vi "表配置.vi"(7 "Item":string, 8 "error in (no error)":errorcluster caption="错误输入（无错误）", 10 "Arguments":string[](array[string]), 11 "数字多用表接口输入":refnum<class "数字多用表接口.lvclass">) -> (0 "error out":errorcluster caption="错误输出", 3 "数字多用表接口输出":refnum<class "数字多用表接口.lvclass">)   [LabVIEW 2020]
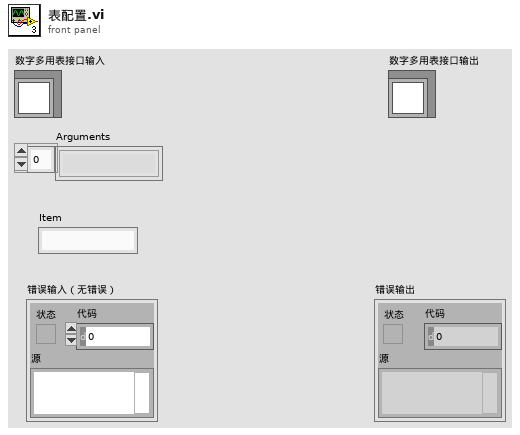
[diagram p1: front panel]
types:
  T1 = enum16{"DC Voltage", "AC Voltage", "Resistance", "DC Current", "AC Current"}
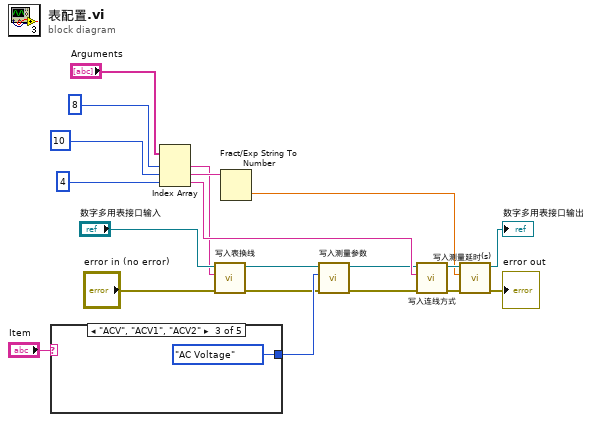
[diagram p0: block diagram]
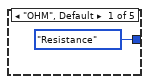
[diagram p2: hidden frame]
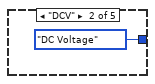
[diagram p3: hidden frame]
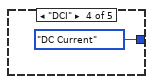
[diagram p4: hidden frame]
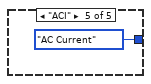
[diagram p5: hidden frame]
diagram:
  n1 = case shown="\"ACV\", \"ACV1\", \"ACV2\"" "Item" {
    tunnel: [T1."Resistance" ("测量参数") T1."DC Voltage" ("测量参数") T1."AC Voltage" ("测量参数") T1."DC Current" ("测量参数") T1."AC Current" ("测量参数")] -> w13
    frame "OHM", Default {
    }
    frame "DCV" {
    }
    frame "ACV", "ACV1", "ACV2" {
    }
    frame "DCI" {
    }
    frame "ACI" {
    }
  }
  n2 = Index Array(array="Arguments", index #1=8 ("索引"), index #2=10 ("索引"), index #3=4 ("索引")) -> (element #1=w4:string, element #2=w7:string, element #3=w15:string)
  n3 = call "写入表换线.vi"("error in (no error)"="error in (no error)", "表换线"=w4, "数字多用表接口输入"="数字多用表接口输入") -> ("error out"=w12:errorcluster, "数字多用表接口输出"=w16:refnum<class "数字多用表接口.lvclass">)  [unwired: 7 in]
  n4 = Fract/Exp String To Number(string=w7) -> (number=w6:dbl)  [unwired: 3 in, 1 out]
  n5 = call "写入测量参数.vi"("error in (no error)"=w12, "测量参数"=w13, "数字多用表接口输入"=w16) -> ("error out"=w10:errorcluster, "数字多用表接口输出"=w11:refnum<class "数字多用表接口.lvclass">)  [unwired: 7 in]
  n6 = call "写入连线方式.vi"("error in (no error)"=w10, "连线方式"=w15, "数字多用表接口输入"=w11) -> ("error out"=w9:errorcluster, "数字多用表接口输出"=w8:refnum<class "数字多用表接口.lvclass">)  [unwired: 7 in]
  n7 = call "写入测量延时(s).vi"("error in (no error)"=w9, "测量延时(s)"=w6, "数字多用表接口输入"=w8) -> ("error out"=→"error out":errorcluster, "数字多用表接口输出"=→"数字多用表接口输出":refnum<class "数字多用表接口.lvclass">)  [unwired: 7 in]
